vi "ACK.vi"(8 "error in (no error)":errorcluster, 11 "Instrument in":refnum<class "Instrument.lvclass">) -> (0 "error out":errorcluster, 2 "ACK":string, 3 "Instrument out":refnum<class "Instrument.lvclass">)   [LabVIEW 2019, in "Instrument.lvclass"]
doc: "Send \"ACK\" command to remote Instrument to test connectivity."
uses:
  Instrument.lvclass
  Typedefs/Instrument.Commands--Enum.ctl
  197db2da-96b6-4d1b-817a-5f02aef6b1ee.vi
  197db2da-96b6-4d1b-817a-5f02aef6b1ee.vi/ea6762b4-f2af-45d9-a79a-86d237a27915.vi
  197db2da-96b6-4d1b-817a-5f02aef6b1ee.vi/be4b8c69-094e-46e4-ae1e-c9a23f2c522b.vi
  <vilib>/Utility/Data Type/Get Type Information.vi
  <vilib>/JDP Science/JSONtext/JSON text to Variant.vi
  <vilib>/JDP Science/JSONtext/LVClass Serializer/JSONtext LVClass Serializer.lvclass
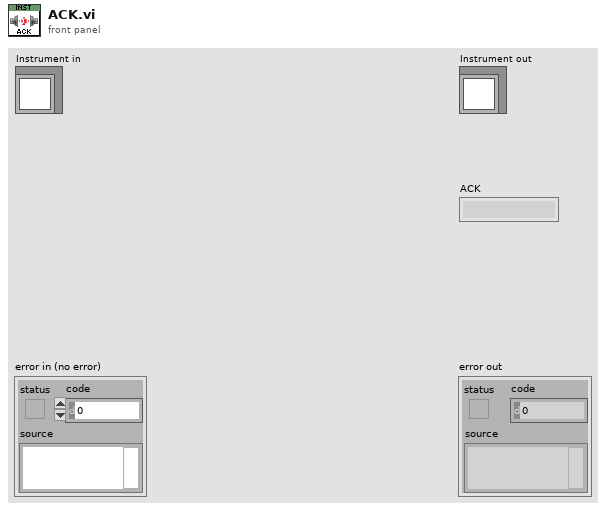
[diagram p1: front panel]
types:
  T1 = typedef "Instrument.lvclass/Instrument.Commands--Enum.ctl" = enum16{"ACK", "HELP", "setConfiguration", "setLogData", "getAll", "getAllData"}
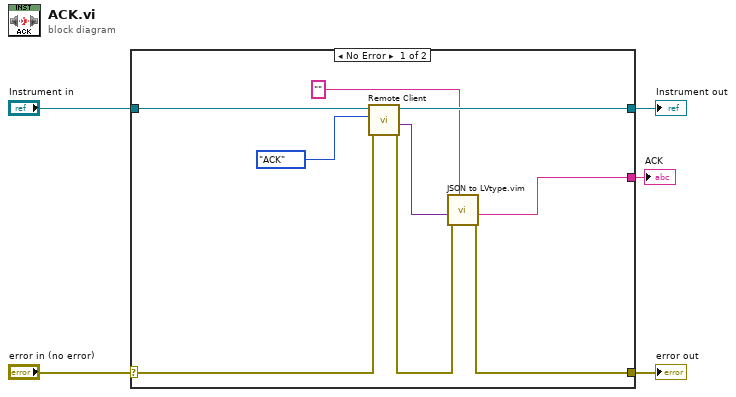
[diagram p0: block diagram]
diagram:
  n1 = case shown="No Error" "error in (no error)" {
    selector: "error in (no error)" -> [w12 w16]
    tunnel: [w6 w16] -> w4
    tunnel: [w14 w15] -> w2
    tunnel: "Instrument in" -> [w13 w15]
    tunnel: [w8 _] -> w1
    frame No Error {
      n2 = call "Remote Client.vi"("error in (no error)"=w12, "Command in"=Instrument.Commands--Enum."ACK" ("Commands"), "Instrument in"=w13) -> ("error out"=w7:errorcluster, "Data out"=w9:variant, "Instrument out"=w14:refnum<class "Instrument.lvclass">)  [unwired: 5 in, 1 out]
      n3 = call "JSON to LVtype.vim"("type"="" ("Commands"), "error in (no error)"=w7, "JSON Data in"=w9) -> ("error out"=w6:errorcluster, "Data out"=w8:string)  [unwired: 7 in]
    }
    frame Error {
    }
  }
  "error out" <- w4
  "Instrument out" <- w2
  "ACK" <- w1
